vi "Configure Profile.vi"(0 "VISA resource name":refnum<visa-resource-name>, 1 "Unit Address (1)":i16=1, 2 "Action (0: Create Profile)":u16(ring) items=["Create Profile", "Delete Current Profile", "Delete Step", "Start Profile", "Delete All Profiles", "Rename Profile"], 5 "Profile Number (1)":i16=1, 7 "Step (1)":i16=1, 9 "Profile Name (PROFILE1)":string="PROFILE1", 11 "error in (no error)":errorcluster {"code" format="%.0x"}) -> (4 "VISA resource name out":refnum<visa-resource-name>, 15 "error out":errorcluster {"code" format="%.0x"})   [LabVIEW 2010]
doc: "This VI creates, deletes or configures a profile."
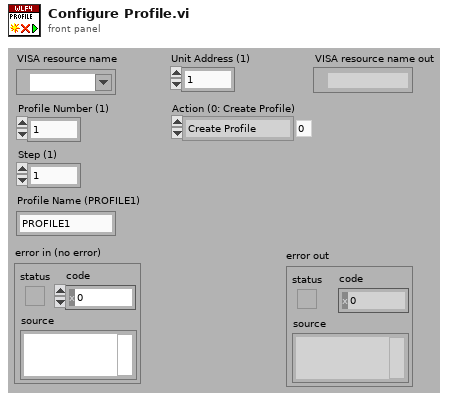
[diagram p1: front panel]
types:
  T1 = cluster{"Status":bool, "Code":i32, "Warning Message:":string}
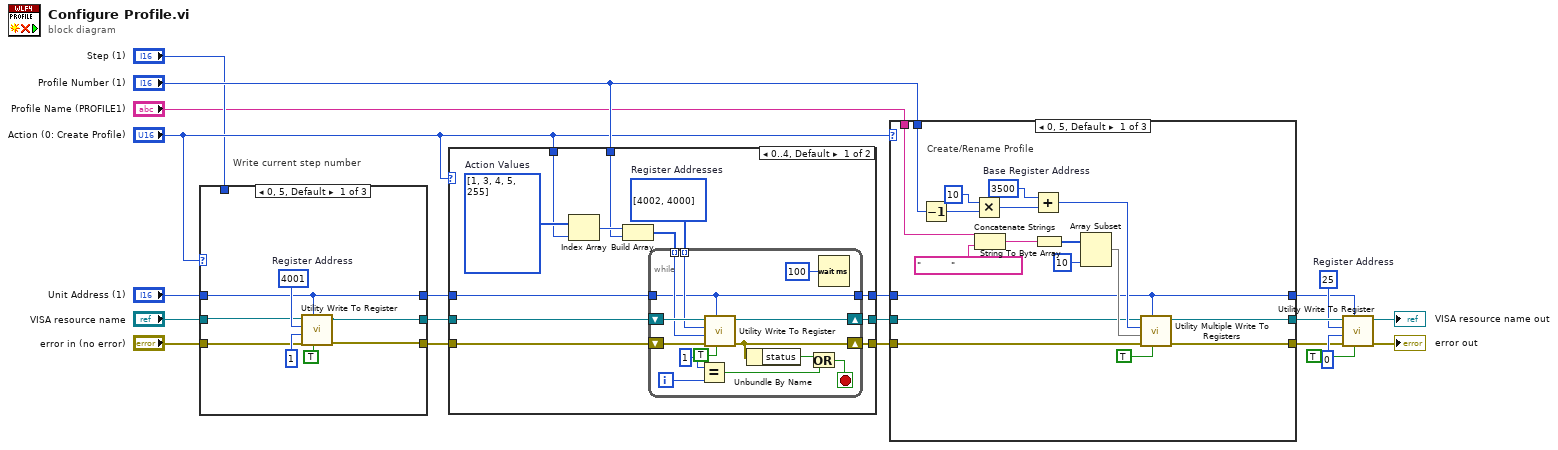
[diagram p0: block diagram]
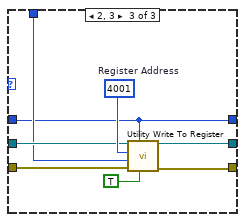
[diagram p3: hidden frame]
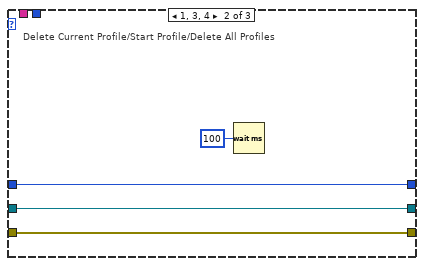
[diagram p5: hidden frame]
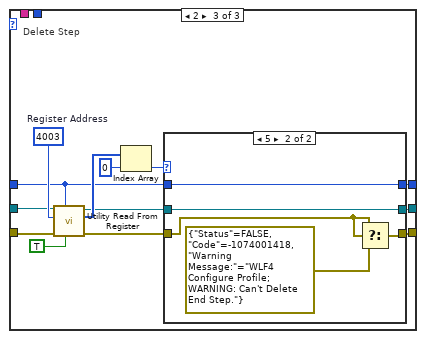
[diagram p6: hidden frame]
diagram:
  w17 = u16 25  # Register Address
  # "Write current step number"
  n1 = case shown="0, 5, Default" "Action (0: Create Profile)" {
    tunnel: "Unit Address (1)" -> [w24 w32 w34]
    tunnel: [w24 w32 w34] -> w11
    tunnel: "VISA resource name" -> [w23 w31 w39]
    tunnel: [w25 w31 w35] -> w9
    tunnel: "error in (no error)" -> [w27 w30 w37]
    tunnel: [w26 w30 w36] -> w7
    tunnel: "Step (1)" -> [_ _ w38]
    frame 0, 5, Default {
      w29 = u16 4001  # Register Address
      n2 = call "Utility Write To Register.vi"("Direct Action?"=TRUE, "Unit Address (1)"=w24, "error in (no error)"=w27, "Data (0)"=i16 1, "Register Address (0)"=w29, "VISA resource name"=w23) -> ("error out"=w26:errorcluster, "VISA resource name out"=w25:refnum<visa-resource-name>)  [unwired: 4 in]
    }
    frame 1, 4 {
    }
    frame 2, 3 {
      w40 = u16 4001  # Register Address
      n3 = call "Utility Write To Register.vi"("Direct Action?"=TRUE, "Unit Address (1)"=w34, "error in (no error)"=w37, "Data (0)"=w38, "Register Address (0)"=w40, "VISA resource name"=w39) -> ("error out"=w36:errorcluster, "VISA resource name out"=w35:refnum<visa-resource-name>)  [unwired: 4 in]
    }
  }
  n4 = case shown="0..4, Default" "Action (0: Create Profile)" {
    tunnel: w7 -> [w51 w69]
    tunnel: w9 -> [w50 w67]
    tunnel: [w49 w69] -> w21
    tunnel: [w48 w67] -> w20
    tunnel: w11 -> [w44 w68]
    tunnel: "Action (0: Create Profile)" -> [w43 _]
    tunnel: "Profile Number (1)" -> [w42 _]
    tunnel: [w41 w68] -> w14
    frame 0..4, Default {
      w47 = i32[] [1, 3, 4, 5, 255]  # Action Values
      w52 = i32[] [4002, 4000]  # Register Addresses
      n5 = Index Array(array=w47, index=w43) -> (element=w46:i32)
      n6 = Build Array(w46, w42) -> (w45:i32[])
      n7 = while {
        shift-right: [w64] -> w48
        shift-left: w50 -> [w66]
        shift-right: [w62] -> w49
        shift-left: w51 -> [w65]
        tunnel: w52 -> [w56] mode=indexing
        tunnel: w45 -> [w55] mode=indexing
        tunnel: w44 -> [w54]
        tunnel: [w54] -> w41
        i -> [w58]
        stop <- w60 stop-if-true
        n8 = Equal?(x=1, y=w58) -> (x = y?=w57:bool)
        n9 = call "Utility Write To Register.vi"("Direct Action?"=TRUE, "Unit Address (1)"=w54, "error in (no error)"=w65, "Data (0)"=w55, "Register Address (0)"=w56, "VISA resource name"=w66) -> ("error out"=w62:errorcluster, "VISA resource name out"=w64:refnum<visa-resource-name>)  [unwired: 4 in]
        n10 = Unbundle By Name(w62) -> ("status"=w61:bool)
        n11 = Or(x=w61, y=w57) -> (x .or. y?=w60:bool)
        n12 = Wait (ms)(milliseconds to wait=u32 100) -> ()  [unwired: 1 out]
      }
    }
    frame 5 {
      # "Rename Profile"
    }
  }
  n13 = case shown="0, 5, Default" "Action (0: Create Profile)" {
    tunnel: w21 -> [w77 w90 w93]
    tunnel: w20 -> [w76 w89 w94]
    tunnel: "Profile Number (1)" -> [w72 _ _]
    tunnel: [w75 w89 w98] -> w19
    tunnel: [w74 w90 w97] -> w3
    tunnel: w14 -> [w73 w91 w95]
    tunnel: [w73 w91 w96] -> w13
    tunnel: "Profile Name (PROFILE1)" -> [w71 _ _]
    frame 0, 5, Default {
      w79 = i16 3500  # Base Register Address
      # "Create/Rename Profile"
      n14 = Decrement(x=w72) -> (x-1=w82:i16)
      n15 = Multiply(x=i16 10, y=w82) -> (x*y=w80:i16)
      n16 = Concatenate Strings(w71, "          " ("string")) -> (w85:string)
      n17 = Add(x=w79, y=w80) -> (x+y=w78:i16)
      n18 = String To Byte Array(string=w85) -> (unsigned byte array=w86:u8[])
      n19 = Array Subset(array=w86, length=10) -> (w84:u8[])  [unwired: 1 in]
      n20 = call "Utility Multiple Write To Registers.vi"("Direct Action?"=TRUE, "Unit Address (1)"=w73, "error in (no error)"=w77, "Array Of Data"=w84, "Register Address (0)"=w78, "VISA resource name"=w76) -> ("error out"=w74:errorcluster, "VISA resource name out"=w75:refnum<visa-resource-name>)  [unwired: 4 in]
    }
    frame 1, 3, 4 {
      # "Delete Current Profile/Start Profile/Delete All Profiles"
      n21 = Wait (ms)(milliseconds to wait=u32 100) -> ()  [unwired: 1 out]
    }
    frame 2 {
      w104 = u16 4003  # Register Address
      # "Delete Step"
      n22 = call "Utility Read From Register.vi"("Direct Action?"=TRUE, "Unit Address (1)"=w95, "error in (no error)"=w93, "Register Address (0)"=w104, "VISA resource name"=w94) -> ("error out"=w99:errorcluster, "Data"=w103:i16[], "VISA resource name out"=w100:refnum<visa-resource-name>)  [unwired: 4 in]
      n23 = Index Array(array=w103, index=0) -> (element=w101:i16)
      n24 = case shown="5" w101 {
        tunnel: w100 -> [w107 w111]
        tunnel: w99 -> [w106 w108]
        tunnel: [w107 w111] -> w98
        tunnel: [w106 w109] -> w97
        tunnel: w95 -> [w105 w112]
        tunnel: [w105 w112] -> w96
        frame 0..4, Default {
        }
        frame 5 {
          n25 = Select(t=w108, s=w108, f=T1 {"Status"=FALSE, "Code"=-1074001418, "Warning Message:"="WLF4 Configure Profile; WARNING: Can't Delete End Step."}) -> (s? t:f=w109:T1)
        }
      }
    }
  }
  n26 = call "Utility Write To Register.vi"("Direct Action?"=TRUE, "Unit Address (1)"=w13, "error in (no error)"=w3, "Data (0)"=i16 0, "Register Address (0)"=w17, "VISA resource name"=w19) -> ("error out"=→"error out":errorcluster, "VISA resource name out"=→"VISA resource name out":refnum<visa-resource-name>)  [unwired: 4 in]
